vi "Debug FGV.vi"(7 "Action":enum16{"Read", "Write"}(ring), 8 "error in (no error)":errorcluster, 11 "RSI Module in":refnum<class "RSI Module.lvclass">) -> (0 "error out":errorcluster, 3 "RSI Module out":refnum<class "RSI Module.lvclass">)   [LabVIEW 2011, in "Modules.lvlib" / "RSI Module.lvclass"]
uses:
  RSI Module.lvclass
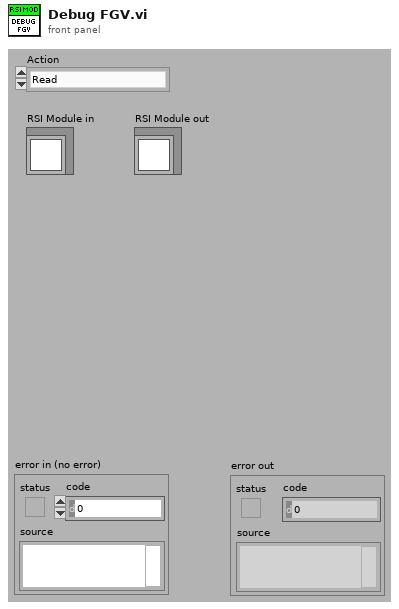
[diagram p1: front panel]
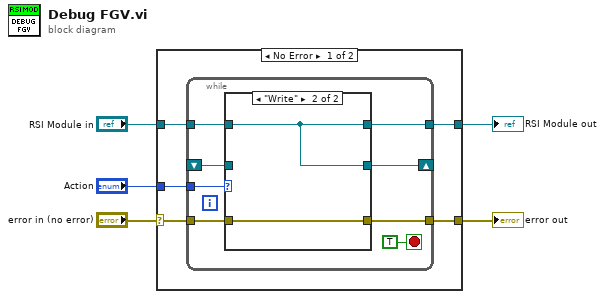
[diagram p0: block diagram]
diagram:
  n1 = case shown="No Error" "error in (no error)" {
    selector: "error in (no error)" -> [w10 w24]
    tunnel: [w9 w24] -> w4
    tunnel: "RSI Module in" -> [w8 w23]
    tunnel: "Action" -> [w7 _]
    tunnel: [w6 w23] -> w1
    frame No Error {
      n2 = while {
        shift-right: [w14] -> _
        shift-left: _ -> [w15]
        tunnel: w10 -> [w12]
        tunnel: [w11] -> w9
        tunnel: w8 -> [w16]
        tunnel: w7 -> [w17]
        tunnel: [w13] -> w6
        stop <- TRUE stop-if-true
        n3 = case shown="\"Write\"" w17 {
          tunnel: w16 -> [_ w22]
          tunnel: w15 -> [w20 _]
          tunnel: [w20 w22] -> w14
          tunnel: [w20 w22] -> w13
          tunnel: w12 -> [w19 w21]
          tunnel: [w19 w21] -> w11
          frame "Read", Default {
          }
          frame "Write" {
          }
        }
      }
    }
    frame Error {
    }
  }
  "error out" <- w4
  "RSI Module out" <- w1
